vi "Main_19A_X1.vi"() -> ()   [LabVIEW 2024]
uses:
  Cluster_Towel Data.ctl
  Cluster_Design Data.ctl
  ENUM_Stripe Select.ctl
  Cluster_Design Towel ID Data.ctl
  <vilib>/Utility/miscctls.llb/LVMapReplaceAction.ctl
  Utility/Universal Utility/TypeDefs_Utility/Cluster_Row-Column.ctl
  9e3f57c0-2ef8-4495-8287-c6a42a5fb955.vi
  Utility/Universal Utility/TypeDefs_Utility/ENUM_4 Directions U-D-L-R.ctl
  Utility/Universal Utility/TypeDefs_Utility/ENUM_8 Directions U-D-L-R.ctl
panel:
  out "Invalid Designs":T1[](array[typedef])
  out "Valid Designs":T1[](array[typedef])
  out "New Design":T1
  out "Design Updated":bool
  out "Current Towel":T4
  out "Current Design":T1
  out "Towel List":T4[](array[typedef])
  out "Target Design":string[](array[string])
  in  "Select Data":enum32{"Example", "Puzzle"}(tab)
  in  "Example":string="r, wr, b, g, bwu, rb, gb, br\n\nbrwrr\nbggr\ngbbr\nrrbgbr\nubwu\nbwurrg\nbrgr\nbbrgwb"
  in  "Puzzle":string="wwubu, guw, uguggg, bgr, rgbrg, bbrb, rwgru, bwgr, uwwbuw, rwrbrgb, ggbrbuur, bb, ugu, grurrr, gbwbwb, rgbrb, bgrwrbu, bgb, wrwu, rwwr, wubr, bug, wu, brwu, w, grbw, uwbgg, gggwrggb, rurgr, uuw, bbw, wbg, bgw, ugw, brb, uww, buww, uuwgr, buu, rrbugw, ggggbgug, wwwrbbr, rgbbr, ugrr, wgwrg, bwuubub, uugg, bbrgg, bbugw, wuuwb, uwr, bugww, rwrrbbr, ugwrrrb, ubbr, rrwbgg, wb, wgr, gbrb, gwgg, rbg, bub, brg, bubr, ugggw, uuugbbb, grbug, rbww, rg, wgwwwwg, wgb, brugbbb, wgrww, bbrgrurg, ruu, brr, grgwg, wurbb, bww, ubwgr, bburwurb, urrrrbb, rgg, wwww, gbgw, rbrb, buw, wur, ruugugb, uwugg, rgrrugub, ggg, ggr, wrurr, bgg, uuru, brbg, rrbb, bbr, gbbu, grug, rwrrug, ggubub, ggrgg, uu, grb, rrrwwbg, ubbg, wgwwrgbr, rbug, rwrgwbrb, wubwgu, rrw, ruw, rbwubwgr, wwugg, bbbu, wgwr, rwgb, ruwg, rrrb, ubw, rwgw, wbr, uwgrb, rbwrrrru, guwbwg, rgbwr, wbu, ubgu, uruug, urbuuruw, rug, wg, gugbw, brw, wgrb, rbwu, wrw, bgggr, rubu, ur, uggrur, ggwbbuwu, gggr, gwu, bbwb, rrru, rubgb, wub, rgb, rbur, wuwbb, rbb, bwb, wwr, wubrwb, bwwwg, wwbwww, ugrrurw, grg, gwuw, uwwww, ubgb, gwr, gwuurgg, grwuu, gbru, rbbrrg, r, rgbrrg, ugrrubr, bw, wwbwbg, brbwbwr, rrrbg, rggb, bgwu, rrgrwwb, wrgrrb, grw, ubu, wgrugw, bbrugug, wubuwrb, gbrr, rrbg, bbg, bgrwg, urwu, uug, gruruwb, bur, rbwrguw, gbbuw, wubbr, gwurrw, rurr, gwrubb, wwwrw, wrwrbbr, ubbru, gbr, rwg, rrgwgr, ugrwwg, wwbgbr, wwubuwu, uwbb, gggbb, bru, uwb, bgru, wgu, gbrgr, urrwb, ub, u, bgrug, rrwr, bguug, gwbb, uuu, brubwg, bwrwbu, ruggur, gggww, rgu, ug, gur, wgurgwb, uuwwb, wbwgr, gbrg, rru, uuwurrr, rbgbw, ubgwgw, wgwbgu, brbwgg, uwwgw, rgww, buuu, uwu, wrgug, gug, rr, gggwb, bgu, grwg, wrwr, uub, gbuwwrwr, bgug, bwg, ubg, urrb, bbgggw, uuurb, ggw, wgrbwrg, bguw, brrrb, gwrbr, brbw, ggrrbu, uru, wrrbg, ubr, ggrr, ww, wwbgwwr, bgrr, wugbrwg, rrrrg, rww, wrbg, ubur, gwb, rgw, bubgbw, gbb, buuuuur, wwu, uubwww, buwg, ugbg, wgrwbub, wurwuu, bbu, wuru, ggu, wguwgr, gbw, gub, grr, rubgw, urrurb, wbubrr, grgwwb, gbwwru, urb, ruuw, urr, gu, bwrbwg, wrr, wru, wug, wbuwwwwg, guugu, brwurrb, brruuw, wuuuu, rbu, gwg, bgwg, rgr, bbrw, bu, gbbg, bbub, bwr, buur, wrgg, wwuurbug, bgbu, ruburubr, bwurbr, rbr, wgw, gwwug, rruu, wubgg, bwwg, wgwbwu, gwrr, wbbrrb, rwbgbbbr, gr, rwuw, rggbur, gbu, uggb, gwgr, guggbuu, gugw, brgww, wuw, rbubgbu, wgwbrb, g, urbb, gb, gbwu, uuug, ggrbbw, wbrrww, wbw, ugb, gbg, ugr, ggwww, rwr, rbrbw, wrg, wwbr, uggu, rrg, gwguuuuu, bbwuur, rgru, bburww, bbbg, wbb, uuugww, bwgg, bgggw, rugbr, wugrbwr, urw, bwu, uur, gggwrw, buwr, rrr, wwb, wgbw, urg, uwgbw, gru, bgbgurw, rwrrgbub, rwrw, buuug, wggbrgw, guu, bruuubw, gw, wuu, rrb, uuuwg, uwbugu, ugbbrr, wr, uw, ruwbw, wwg, ubru, guub, wrrwg, www, bbuuuw, guruub, wwbrwu, rwgbuu, rguruww, bgggrwr, bg, uwuwr, ugwub, ubgbu, ubbur, rub, gww, rw, urrbbbbu, urrbb, wuwu, ubuggww, bbbwg, ubugg, grgb, rwu, rugbug, ugg, wgg, gg, ru, wruw, wrrwuw, rubg, rbw, rwgwr, uuruu, ubb, ggb\n\nuwgwguuguruwggwbrbwurruwgwwwurgbgwggwwbbubgugguuurgugugwu\ngwwggrgbwbbguwgbguubbwrbgurgbburrgbwruwgurgwgguwbwgbgrr\nrgggbwgwgwuubwbwrrbrrrurwuwurgubuwrbwrbbbbr\nrguruururrwbbrgrbgrbwggrubbggbrbrugrgugggurubrbuuw\nrruggbrruruggubguwrubwbwuwgrwrguuurbrrbbbggbrwg\nwbwurbbrggubugbrgrrbuuwubwurrwururgbgbwurubbuuwbuw\nbrbwrrruwrrrubrwuugrbuuwuuwrwrbrrgububwurugbwwrb\nrbbbuurubwubbuguggrgwgwgurburugugwbgbuwbwwrrgugg\nwrbbugrwgwubgugwrruggwwggurrwuugrwrwbrwgrww\ngbwbugwgrubbbbburrbwugbwuugrbbwrrwbgrwubgwgbbb\nurgrwbruurbbururwrwwbbubgwbwurbwguguwgrbrgugugwrburb\nwubuubwggrgwgbgububrwgwbbubgwgbwwwuubrbbbuwbr\nwrrrrurbwubwuuggwguuwwwububrwrruwurrbbbuubggwgrgwugwu\nbrurwwrbbuwgugbruurgrrgbuuwrbwrugurrwrurrrbbwrwbrrgrwuwg\nurgwuwwbwwrbbwbwgwgrrbrwgubbrbgwububbwurggbrgrggbrggrrrwgg\nuugwrbwguuwwgbwwwburburbwburwgwguwggwggwbbbuburrubgbbguugg\nwbwbguuuuubwwbwgrwbwgguguwgbbggwwwurgrwgrgbgggurbuwugwrbu\nuubwuwuuwggbbruwuwbwbgwbwrrguwurubbguwwgbug\nbwwgwwubbrrrrwuubwbwrruurrwwwwggbgbrwububwwurbggwuwbgu\nbruwgrwwbrwbgruubwbbbugwrbbgwguuwguurbrwrb\ngrbgwuwwrbgrwgrwurrwbbuwwwwwbrbburrbrwbuggrgwbwrb\nwgggrubbbwwgwgggwruururugbrguburrwuwwurgggubrbwwgrwrb\nwurbwrwwugrgrgruruuggbbggubwrurbrgrbwwrbrrw\nuubuwwurrrrurubbbrrugugubgbruubbrwbuwugrwwgwrrbrwggwrb\nggbuwrwwwbbrgruugrrbrbuurwgurwgubrggguwbubrrbbwgwrb\nugwgurwrwwbrrbwrrrruwbgrwrurrrrrgugurwbuuubbubwwbgrrrbwrb\nurwrbbrbwgurbuwrgrurgwggubbwubuggrgbuwgurbbwwbbwwubwrurgrw\nbbugbwrwrrrwbgugbgguuwwbrwbbwgurubrgugrgwurrbb\nuburggbrbuurrbbggububwbuuubgwrruugbrrbuuwb\nrrwuwubggwrwruwrgrrwrwubwwrbbbuggbrggurubwubwbuggwu\nrwwuuubguwgwuwgwwwggwbwrubbrguuubrurbwuggubwbruwrb\nruugbuurwwwwrwuwurrrbrubugubwrwwwgbwbrbgbwb\nwrurbuuruwrbwgrbgbbwgwrwrrrwgwrurbrbuwrwwgbgwgrwgu\nbbruguugubrrgrgurwwggwurwbgwbwbbuugwwrbwubwgrwrb\nbbwgrrugwgrbgwbbugugwuubrbrbrbbrrrggurgbbwwuwrbbuwbgw\nrbgbwburggggrbwubbrrrrggbuwbguggrrbuwbgugbbrgwrb\nubgwuwbbgbubrgbububwuwbbbburwurbwbbuburwrb\nbbgubwgruwbuwbwrwrurbrbrubuwbgrugwbbggbwgrwrburguggwwg\nuwuubwuwgbuurbugubbgguburbugugrrwbrrurgwrwgrgbb\nwwuuugrwuwurbgwwbrbwguwugbgrbgwwbgrgbubrrgrbbgwrggwgrwgruu\nbbbwurgwwbwurwubbugrwbwbgbwrbwrwububbgbgurwwruwrwrrggrugr\nbubuwbbwrgrwuggbgrgwbbwruubggubuwguwgrbrrguwgwubbbbubugw\nwbwbguwgbrgwgwrrurwwrrrgbrwubrgwbwguwbwwuwgugwgrbbubgru\nbwbrbwbrbubbwwbgwwuwgwwgggrrgwbubbubwwwugrgwgr\nwgwwwwurwubuugruwbrrguwgubwwbuuwruugbwrubr\nrgbbbwrgburwuwwbwubwruubgguwbrbwbwrwurbggbwbrugwgrubrgbbur\ngguwwggubgrgrgrwuubruuurubrbrruwgrrwrwuwgrwwburwuwrg\nuwbgrrwbbggrwwgguwbbgbbrugruugbgrbuwgbugwrb\nguurgurbwbbrugrbuugbgruwgburwrwwrbgbrrrgbwbuwrb\nuuwuggwrwgbgbuguruwrgbrbrubgrgugwbrugwrgubbrwuwrb\nrwgguuubwrbbrbubbgwwgrgbbrrrgggbururgwgbwgugwgbgbrbbb\ngrwwrwbbruwubgbwuuubwgubguruugubbwggrgurrbwurgubbggwb\nbwuwbggbwbgwbruuggruurrwrwgubbwrrubrwwbgubguwrb\nrbwbbrgrwgbgwgbwrrurgbrwgwurrwbrwwuwrgugrbgrugrgubbwrb\nwbbgwgbwrubuwgurwbwbugwguwwwgbuwgruguwbgbgbuubwuwgwubgrbww\nuwwbwrbubgbwwuwwubbgbgubwwwgwugrgugrwwwgwbubrguggbrgrbrgg\nwbwuwgrwwguwgurwwurwubgwuwugrbbggbrruuwbgurrru\ngbugwgrurugwrrggbrbubrugggwggbubwbwrubububgbwrgwuurugwrb\ngugrgwugubwuwbbbuurrwwrubbwwwguguwwbbruuugbrwwwuwuw\nrwbbgbugrgburrggrgwgubggwwruuggubururggrbwrb\nrgggggrbbrgrrugwwwgwbwbbrrbrburbwbwwrrgrbuugrruwbbuwrb\nubbuurgrwwwuwbwwbgguurbbbgwbuugwgwuggrrbugguruwwrgbgggbbuwrb\nbwuruwwubgubbggrruwgbbgggwrruubgurbrbuuubrgbwub\nrbubbggrbwbgwwrrbbggubwwurwgrgwubgrgrrbwrb\ngwwbgwubrububgwrurwgurbbuuubwugggbrrwuuwru\nwguggrbbbwgrbrwwggrurwbggwgbrgggrwggugbrgwgg\nuuguuwwrguwrrggugbwwgwuwrguwbguwuurbwbwrggwguwrubwrb\nruuubbgrgrrrgbbrbgbrbubgbubwguububuugubgrugbgrgwrgwrwruggw\nruurrbwrbgubbuwggguwbwububrbwgrubbwgugwrb\nbbgbugbrubwggbrrwwuwrwwwwrwbgbbggrrwbguwrbwrb\nbrbugwrwrbwwwguwrgrrrggugwwruwburugurrgrurbguwguwwbrubu\nwbwubgbubwwgrrggrbbgwruwrrugwwrwuuggbuuwburbrugbguwrwrb\nuugbuuwwburgbgruuruguuuwrbwurwggbbwrrbgrurbwub\ngrrwguwurwwuwgguuugurwrgurrwgrgugrurururwrb\nwwrbuwwwwrbbgwgwbgrurburbbwbgwuugbuwuuwwuuwbbuww\ngggrbrwrugrrurwugwgbgugrruwrrruurbwuubbuuruuub\nrwuguwurugbrububbrggrwrwururwuwuwbrwwgurwgrrrrbrururrwbgbwrb\nrwbbgrbbwgbrbbgugggwwububugrbrgwgubbggwgrgrbrrbrgwwuwg\nwururwgrruuwrgrrrwbruubuuwgbrrwbgrrbbbgugbgrrguugwg\nuruwurbgrwrgwbrbbggwwbgwbgwrbrgrrugwbwrwwbggbrgrugwrb\nwrubuwbugurguuurugburubbrgrurgwugwwbbwuwrb\nbwrwgbwwbuuwbwgbwbbbrbwgwrugbubbgubuwrrwguurgrurwwwbwrb\nrrwuuwbruwugwguurgubwrgwgwgburbrwwwgbubwrwrgggrwugurbrrbu\nrrwgrgwwubwgwbrubwurbbrgbuguwbuggbrwrururrubbwburw\nuubrgrrbgguggwrbwbwwwguwugugbbuubgugrrbugbruggrwubu\nuwrrubgbrrgrbgrrrgbrwgwgrwbwgugguwwwgruwbuwwrb\nwbgubgrbrrrwbgrbrwrggugruuguugubbwrrwugbbrubrrbuubbwrbwrgw\ngubggguubrrguwrwurubwwubbugrwugwugguugguugbuwwwwubgwgbwwuu\ngwguwggwgwbrugwbgbgruwbrwgbgrwbgubbbgwgwbggrw\nwwwburgwwurgubugwrubrggbgbrrbgbwgggwrggbwbbbbubrbuuw\ngggggubgburbgrguurbruuruguwubrrrbruruuguwwwgggu\nbggruubuugbbubugwrrbuuwrguggrwrwurubgbwwwbuuuwgubguruw\ngwgbrgburrbbgrwgrurguuwrrwgggrbgbbgwbbbwrgggwbrbrgwur\nwbbbbrggurwuugbruubrbwgwgurbwuwbrbwrbwgruwrwwgrwurwuruwrb\nbbggrguugwrguwbgruwrwbggurbguuuubgrurwbbgurrbgguggubw\nuwrrwbwubbgwbuwwuwurgwurbrruruwuwguggrwbwwurwwurgbgu\nubuubuwrgrwugguuubwwgwrruwwbuwggbbwwrrwbrgbuugugwwr\nrwwbbugwrwggwwwuwwbgwwrrrbggruruburubrrubggrgwrb\nbbgbrwgwrgguwwrubgwbgubuuurbwwbbbbuggbrgbwrb\nubugbuwbrguwwbrgwrgguwwburgbuubwwgbgrbrubgbgr\nrubwrrgurbuwbrggwgbgwbggwuwrbuwgbgubrrrgrrwgbbg\nubrbrrgurwbgbbbrrrugbrwwgwugbrgbugugugrbbggrwbgubbbuuub\nwuwgububguurguugwuwbuwubgruwbwuwbubuwburbgg\nwwrbgwrgwubwrgruuggwbwwbrbggurburgrggubgwrrgrgrgbbrbgwwuuwrb\ngbgrrbugugwrrbuwrubwuwwgggwrbwwrugbgbgrgrrruw\nbwwgwruwugwrgwwburrwrgwgubbrgurgubrwwrggrggbwwgrguuwww\nrbbwurrgrwrbuwruwuwuuwrgugbwrgrgruubwburbrgbrubgrgrwguur\ngwwuurbugbgwuggwwwwwbwgrrbbgrgwwbwgrggrwrbugwrwrb\nugwrbrgrggwbwwuubrwubuuwwurbbbbwgggwgurbggw\nbbwggbubgwwuurbuguruwwbgggurgwbgrgrggwurrrrurgbrrugrgwgww\nuugwuwubrurururbggrrgurwgwgrrgwwgrwurwrwurwgruu\nuwgbwurruruwwuwgbbgwwrrwrwbwgrrbwbrwgwbbwubrgruwub\nguugbrrubwbrbgwrwwrurrwwgbbgwgwrbuggurgruuwgrub\ngbgurwuuwubrrugwrrugwbbbrwbrwuggrwrrugrwbgu\nbwguugwwwuruguwrrwwbbuguugbggbwbubbwgwrgbbguguruwguwuru\nbbwrbrguwrwbrgruguuggbgrbrruguubbuwwgrbbuwrwwgrbwb\nbuwbwbbrurrbubrwgrgwwwbgburbruruwbbbubwrbuuwgwwbwu\nurgrrrurgwrggugwbrwubgguguuruurubbwrrrwrb\nbburwruuwbugrbwruuuwguubrbuwuwbgbgrbubuwbgr\nrbgrugguurbrrbbwruuuuwgwrggwwurbbrggwrruuuurgggbrbrbrb\nrguwurugbwbwrbbggrgbgrgbwwuwrbbubugrwrgrrrbbbrburgubgurggwrb\ngwuwuuwugwgguubruwwrubrurwrgwrbbgruuuubwwurrugwuuugwubg\nbgubgwwbrbrwruugbbbbbwrbguwbgwgubgbbgbbgurgrurgggugbbwbr\ngruwwbwwgbbwwbwgwgwwubwwbwubwrwrgurwuwgrbbrurgwg\nguguwggbbbgbggbrbrgwbgbrwbgrgruurwurbwggbuwug\nrbrbbuurgbgbgbgggbrrwuwuwgwbwbwwuwbgubbbbwr\nbgbuwugbugrwwwwgrbbgguwbrbwuuwgrgggrrbgwbwgruggggwwubbwrb\nggwuurgbwurbwubbrgbbubgrwguwbrwbrruwgwgbrwgrrurggwub\ngggruuubuwrrugggruuguubbrbbgbruubuwrurwbrwggbrgrrburwggw\nrrugwrwbrgbbwrgwgbbbrwrgbburubggugrwggrbrbwubrgurgbwrb\ngrbrubguwruuwggbwugwwgwuwwggubuwuwwrggbrbuurwubwbbwrb\nuwbwuwwbbrguburrwrugburgrwuruwugbburubwguugwwru\nuuwwrubggwwwuugrgwbwgbbwrrbburuguurbrbwuwwrbggurbbwguuw\nubugbwrguwrrwurwuwbrbbubbbwbgugwgbrbwruwwwrububgur\nggrrburgrgburuwrrubububrrbgruuguuuwwwgwwrgbruub\nggbuugwurgbgrwggurugubwggbbbubrgurrwwburuggrrrgbbbbwg\nggbrgrwuuwwbwbuwwwwgguwbbuwuwuwuwrwgwwubwwuwrb\nwrbrgugwrbwrwguggrrggbguwrguuwbwwrrubgbbbuwwrrbrg\ngbwbwrgrbwurwuggwwrwwgwrbbwrwwrbrrrrbuwuurrburruu\nbgugggbbburbbbrguurbgrugwwgggurugbuubuugubwrwr\nwrgbrrrbwwurbgbgbwbuuwbwwbugbgbugrwgwuuubugwrggwwbbbwggwgwrb\nwwbwbbrwrbruwrurwurwggwwbrbuugbugbrwgubggrr\nbrbubbburuwgrbuwwuwrurrwwubrwugwbgburgwrggbwuwrguwgwuu\nrwurrbrggrrgbbgbuububrrwbguwrgbwruwgrrruburuurwwrwbuwgbbr\nbwggbuggrwuubrrwubuwrgwrbuwwurugrbbguuwrrugbgburggububww\ngruuwburbbgbrbwgugwgwuurgububuwugguwuwwrbw\ngrrbgwbwrbrwgwrwuugwbbgrrggggwuwgwugbbgugwbrugwbwu\nrugruggwruburugwugrgwbugwwugwuwrrgrgrggubrgbwgwwwg\nurubrbgbgrgwwgwbrgbbwbrruuruuruuururggubwr\nburbwguggwrggrwggubuurrgwbgwggwrugwwuubgrbwbgrrbug\nwwbwgrrwbwwbrugrbgwgwgrwwggwbrbwbgggguuubwbgbburguggub\nurrbbbburgwbwbbwrgubbggrwbbubuwrgggubggwrb\nggugrbggurrbggrwruwgrbrwgwbuurrgrwwwgugurrrbwgbbrbbggwrb\nbwgubwruwrgbrbwgbwbbgbwbgrbbruubbuugwburwrb\ngwrbbrwugurrbugrbgruwruwrwwguwubwubwbrwgrruggrr\nrwgubrrugrwwwubrwwwrbrwwrbgruwgrubbgwgrwrb\nbrrbwgwgwggugbgrrrrgggubbwwwuururbgbrwugwbrbrbwuuwru\nurbrurgrbgguguguuruwurgugwwgrubggbgbwwwgrbugubwggr\nrbgruguwrurwbgwgurrwrrrggugrwwbrbrbwgubuwubruubwrurrgwbgbwrb\nggbwuuuwggggrububwwrurgbrbrubbwgbbbgbbbgbwuwwgggbwrbuwrb\nrbbbburwggwurrrrbggwgwwrurubwbgbrbruguwwrwrgggrugubw\nrgwgwwrgbrgrwgrrbrburwbwuugbgrwwwggrwrbbwrb\nubgrwwwuubwwwwgbbrurbuuruuurrbuwggbbuurgrrwrgwb\nwgwwuruurbgwruugrwgrbugrbbwbgwwgguubrwrrbr\nbwrwubggwgrrubgrrwuwuuugruuuubuwbrbbwrrbgrwugwgwugrguwrb\nrguwgwugururbwwgwwwgwgwbugubbrbrgwrwgguguwbwruwrrrbgbu\nwuuuugurbwrgbuugbrrwgggwwwrwrrrrgwrwggwrbb\nwwbwbugrwbbuwwwrwrrrubrbgwwwburwgbgbwwbuwrwugguurbg\nubgbuubgrrwruwugwbwbwbwwgbwbuurwwuwbubwrbug\nuubgrgrrugubggggwgrbgbrwrwbrgrwbbwgrburrbr\ngbwwugwbgggrbguurbrburbwwrugguwbugwwugbuwwbguu\nwuwgrgrgwgrbuwgrbgburuuwrbwguuwuruwgbwwubwwbururbw\nwwrwgugurwrbbbrwbwubggguuwrwbuurbwbwubggbbuurrwwbubuwrg\nbburgruburubrbwrwwwbrgrbuwgwrwggurburubrgwgbbruw\nubrwbwubbbbwbwgruwuuwbrgbuwwuwuurrrwrrrwgb\nwwwwrbrrguwugugbgrggrubbrgrurggbgbuwwbrgggwuguwugbrwg\nrbrbbuwrubbbugbgwgurggrgbwrrurbburwrwggruwrubgbgwwuuu\nwuuugbgwgggburrrrgwbubbbgrubbgburwrbugbbwbwggrgrg\nrugwgubuwurrguwbwwurrggrgrurgwbbwbubwwgbgrubruuuwwbu\nbgburwubrrwburrbwgwuwwwwurwuuwbgbgrwggubuwubwwggrwrb\nuurbururruggwrwuwbguwwwbbwrbbwrggwrgbwwugwrwuwrw\nbburugbugwwwwggggwruwwggrwwrbrrbwgbbbuwgwgbwwwubgrgbwrw\nrgggubrrbgugguwwuuwurgubgwrbuwubwburwuubrgb\nrwrgwbrbbwrbuwwuurgwuwwbrbrwuububrgubbrbwrguruuub\nuuugrguwruwwuwuuwgbbrrwwgruuwbbgwguwwruuwrb\nbubbubgwwuurgwrbuuurrwrwwrurwgbwugguwgbbggggww\nuwruwuguubrrbbggbgrbwrwwwbwwwggggruuuguuugbwrwwrgw\ngururwuubwbbugububgwugbugguwuwgwrugbrwrwrb\nwrrbwuuwbwbubgwrruwgguwgrbggubrgbgugrrgrubwwwbwbr\nrbgwbgwububrrrwbuwwwwgrurwrbwrgurwruggguggurrrubbbwrwgww\nwggbrggbrrgbrrgrggwbbwurbbrgugugrbrgrwwbrgubwrwuuruubwugwrb\nrrgbggurbrwuwrgrbbwwubguwgurugurwurwbgwrrbbwwuwwbg\nwbbggrwrgruwgrbrgburwggrrbbbguurgubbuwbruwwrggrbr\nwubugrwrrwuuugwuubgrubbbbgurguwgrwgruwwruguburwuwu\nwbwuggubbrwugwbwrrwurgubuurrrubrgwbruugrgbrrbrugbwrruwuubwrb\nrrbuwruwguburwgugrwgwuguwuubgurggrbuugbuwrb\nwrrbuwggurrggwubgwwuggbwuuwwurrrwwrwurrburgwbwugrgbuwwrwrb\ngrrurwggwgruwrrbbwuugrwgrgggbrgubggbugugrwrb\nwwwrwbuuwgbugbwurrgwuwbuuwrbuurugurwbuuuburrurwrb\nruruggbgwbggrwwrwrbrrgwuguwwrwurrguwugurbbruwbrwuu\nuwuuggwurgbwrrrbruwrrwrurgrwrbrwugrwbbburwurbwbru\nrrbwuwgrwuugwguugbrwgubrbubgguwrugrwbwrrbggbgrrrugrbbgr\nrgggrbugbubburuwwbrrrbuubrrwubuuuwgbgguuuurrubrwwuwwugrbwrb\nurrgwwwrgwrrgurrgwbbrggwrgubwgwwwugruuubuuwggbuur\ngbuguuwwrbggrwrrubwwgrbwrurugrwrguuuugwgwrrrgubgbwb\ngwugrrwrgubuwggwrrguubugwrbururwgbwgbbugwwwrb\nbruuwuwbgrbrwbwwubrbbwrgwubgggwugbuwgbrwbbwruubgwbbrwwwubg\nwwgurbbbbbwbwwrwguwbrururbwurgbgwurrurbgur\nwwrgwuurruwuwugbbrwbwrbbbuwgwwububrwwgggbguwrgwrwrrub\ngugwrrrwugugruuwrguwbwwubbggrwbgbwrugbuwrb\nrgubwgbggwbbwggwgggrrrgggbuwwrgrwggggrrgwr\ngbgrbggbgggggbgugwgubggwrwwwrwgrbrguwuwgwrbbrbuwwgrwuwrb\nwwbgrrggrbgrbwbrrrbwrwrwbwrbrrwbwuugggwrb\nwbbwbwbgrbwwwuguubbwgugrugbbrbbggrwwurururwggw\nuguwrggruugrgwwuubbrbbbgbbgugurruwruwbugwrugubwwbgbwg\nruwbwbrubggruwbrwrurbrrrbgrrwrrgbubbrwrwurwuubwbrruburwuwrb\nugrrbgbbugruruwbgbbbgwbuwgbwugurbrwbgurggbubwwrbb\nwbbwrwrwgurubwgbrgwgrgggrguruubburrubwugggrrwgbbrugw\nuugwubrgwuuwbrrrbgruuwruwwbuuubgwuwwwuwbruguuuwgrbrwrb\ngugubrrggwbuugubrbgwgbubwwgrrurubwwrbbwbrgrr\nwrggwguuguuwbgburwwgwgwbruwrgrrwuwwrgbgugurwggbbg\nwwuugbgggubwwwgrgrbguguwgwwwgbuwgbugwgwwguwrug\nuwuurugbwgbrrbgbbuuwuggbrbrwubwbrggwbgrubbrrggbuubu\ngwggubgwgubguwrbggbwwgbuurbbuubuwwugbubwbgbbruu\nbbubugbuwwgbgubrbrguwggbbugggbuwuubbwgrwgwg\nrrrrwugwuurrrbggrbwbrbrugbrbubugrbubbrguwwwwwrrgwgbuugbu\nwrurguruugbwrwbgguggbwruwgbbwgguurwbgubwruuwru\nrwbbwbrbwuwrubgbgwrbbuwbgubrgbwrrwwuwgbrwgurgubburuug\nggwubrwwuggrrwbuuubwwgbbgwurwgrgwwuwubbrgruurugwuguggurg\nbbrugurbrurbgrbubwurrubbrbbgugwbbbwuuuwrb\nwwgwwbruuuruwggbbwuuuubgwbubrbgwbwwuruuguw\ngburwbwbgrbwbgrugbuwubgrrbrrggbuwwrwrwbguuuu\nuwuwgrbggbrwgwggwwgbrrwburuuguwbbwwwrgurbgurrwgwurguwrbwu\nrbwrbuwrwgbbwwggrbwbwwggrwguwggbwrgbrrubgubgugwbrruwwrb\nbbuggbgbwgwrrrggbubrggrurugubuwbwuguwbugrrggwuwbwrggbwb\nugggrbwgwuubwwggggwuwwwruuugrrguwwbwubrrwugwrrurwgbg\nbwgrgbubgbuurggguubwwrwgbubgrrgrgugwrguwruwbrbwrwbbwbbbb\nwrrrbgrbggruggbbuwwuubrruwgbuuubgwbguurrubbubb\nrbwrrrrubruuwgrgrbgwwwurwurgwbugrbbwwgggugbu\nugbggrgrguwwwggbruuruubwwgbwuggwbrwbwwbrbwubrubgbrrgwuwrwrb\nrwrbrubwbburrurbuwgrrrgurwgrwbrgwgwwrbwgbrwr\nwbwrbruubggrgwbbrbgrbuwwrrrbwwburwgwguubuwguwbrgubbwrbrbwrb\nrgrrbwrgwbbuuuruuwbrubbbuburguuburrbgrwbgruwru\ngwrgrrbubrwgurwgruwguurgruruubgubguggbbwwrb\nwgbbuwurburbwwurgbgbwgggruggwurbwuwbubrwrrwbburbgrwgug\nubugbggwuwguwwwuwugwbwgwwuuuggrrrrubwwubwbwrwrrugwbwrgwuu\nrubggguguuwgbuwggrruwrwrgruruguurrubwuwrgruwwgrrurbwuw\nwurbburwrubbwbwrruwrbrbuuugurbwuwwgrbrbggwwbgugubrrg\ngugruugwruwuwrugbgurguguuwwbbrwrurrgubwbwbrgbwrb\nwugrbrbgwbbuuwrrgrbwgwrruuuubrbruwggurgbrg\nrurwugugguurgubwbuuuurrrwbrrurbwruurwugrubrgubwrub\nrubgwwrrwwwgguuggbwuruwwggbrubwbrwgubrrgrwwbuwggbbburwurbwrb\nwbbbggwuwbwwgguruwguwbugwgruwwrwrgggurwwuwbbwubgu\nbgbwbbwruuugugbrwburuwwrwbbbuggugbwubrrwgwugbwguguuuwru\nrbrwwwwwgbruwguuuuubruuurgbuubrwbrbrwurgburbub\ngrruruwbrwwrbgrgbgrwuwrgwwuwbbwgrrrrrrrrrggbbbwbbbbu\nurrwbbbrwuggrggbgububbrbubuwggwuugwurbbbwbbrwrb\nrwwubggwrrbuurwwrrruuuruwggggwbbuwurrurugg\nbgrbrruwrrgrwbwruwbwbguugbrrggrbgububwbuubrububggugg\nrwruuwbuwruuwrrwgbwwrbwwwbwwrwwuuggbggwbbrbbbwwg\nrrgwrgwubgwrwugbuurgruburburuwwwbwwwwrgwwrgwrgrgg\nwgwrrgwwurrrubwgwrgbrbwgbbubrrrgugwwguubuwrbbb\ngurggwuurwwurwrggugwugrbwubggwwwugrbubwrubbuw\nuruuwurrggwbgrugrrbbubwbwwggbuuugwgrwbuuuugrrwbr\nwbbguguuwuubwwrbrbbrugwrwuuwgrggbbwurrubrrgwwrb\nrruuugbgbgrrwwrwgrbugburbubuuggurguugbwgggwrwwbubb\nbrbgwwbgrugurrgurbbwbrwubbrbrrwugwrwugrwwrb\nbuurubwuubrwbugwbbrrgwbgubrggubwurggwbrwwrrurubwrgrrg\nwbrbrrrgrrbwubwgrwubgrgrwuubbgwwwugbwruwugwwgubww\nuwrgbrubwbuubuurrrbwuguwbggurbubuwgwbwrggbggbwruwuggguwbw\ngwbwgbwbgrwbgbbbrwwggbgrurgrwguwgrbruuwbugwrbuwwbwrb\nguwbwbrwgbgrrrbbrbruwwbbuwwggbwrrbuubugwbrwrb\nwrubrurubbbuguurrbguugwurwuuuwgubrwbbgguwwbbbwwwrbwgwuwgr\nrurgbrrbwwbgwbubuggwugrubbgwwwrubuuwbgwgbgwugrrugrub\nrwugwrwwbuggwbugbbwrbwwruggbgrwuugruurgrbwwbuwwurubgbr\nbwbwuuubbgurgrgrbggrubuuwrugwgwuwggwrggbrbwubwgwguwwrb\nurrgurwuwwggrubgrrwrugbbgbbbgwrguggrbuggrgrgwrb\nwuwurrrrwbwgwwggurwuwbrrgrburggbwgrggbgrbrrggburrggwwrb\nubugrbugubbwgbbbwwgwgwgbguwwbrgbrgwubbwgwwruubgrgrrrb\ngurwwrggbbbburwbgububbrwrggbuwgbwrbrrugburgrgbu\nubgbbrrbubrrubbggrbgwbwrbrwubwuurgwbburwwgr\ngwbrrgwgubbbbrrubwgrguguggwwrbggrwrwuuururwrwguwgrbuwbuuwrb\nggbubbbbwruuggrwwuuwbbwubgbururrggrbbwgwrb\nrgbbrgrwgrruwrwbuurgugbrububrugbgwruwbrurbrwwuwbbrgbbrugr\nurruuurggrwgugbgrwgubrbbbbwuwrrwgrubrurgrbuwrgwu\nbbwwwwrbbuwubgrrgurbbruwrbrwguwrbwrurwwwbbuwgruubwwwrb\nrbrggubbuwguwbggbrrbbwrrurrrbuuuggugububbbbwrrwb\nugwgwwwrwruugwrwrbuggwuuwgbubwgrbrwwgrggrrgrbrbgbbwgwrb\nggugburbbrgrrwgwbwbwruuwugrbrrrurgwrbrrbrwubr\nububbrggggrbruugrubrwrbgbwggwrbrwubggubgggrrgbubrrgrwrb\nrrgwwwrugrurwuggggwrbbwugwwwwububgbrbguwwwguwguwrb\nuuwwwrbgrrbwgwuwrwwwgwwwrbbrbuggwwuguurwgwrb\ngurrrubbgwubwuggrrwwbbubbrgbgubruwrgubggrwgrburrrrg\nuwugubuuwurruwruubgbgbwwggbrwgwgrbbuwugwrb\nwwwrbwrbwwgbrbrwbrggrgwrurrbrbwuruuburbubguwwugggrbwgwgb\nwbgugurgwrrbbwugwbrwuwrwruruwrrugrruugwuggggw\nrwbrwwgrgwwgrwgwbgwrwrwguubuwwbguwggubwggwwbww\nrggrruwggwrrgggbrruwrgbuggbbgbwbwgurwrugwbgwwwr\ngbbwrgwwrwgguurbggrbgbwggbbbuuwururrgrgwgbgg\nwbgruwwwubrbugwbuwuubwgrubguwgwbrubrgwwwgwbgwwrrugbgbub\nugbwugubwgwbuggrurguwwubwrrurrbrgurrbrubwuwrwwwwwgwwgrwwbw\nwrwubuguggbrrbugwbwwwrguuuguubwuruugwbgwbguurgwwbggrwwbuwrb\nuuugbgrgwrugwguuuuurwgggrburwwgbwrurwbgrrwrb\nwbgwguuwbbuwggubrrwbgrgbwuwrgbubruwggbrrubbwg\nubuwbrwbbbwbguuwgugrbuwwrgugwubgrburbgbbrrgrubbbbbu\nugbubrurbgwgwwgrurbwugbwwwbbgbugbbbuggrwgrbugbgwwbuwrbuwrb\nwgrwwuugurbgrrgwwbwrubrgrrwwubgbuggwbbuwubu\ngbuwrwbrrrwrwbwwrgbugrbugbrurrgggrgwgwgrrbgubrr\nwugbuggubuggbrggubwgggbgbgbgurrgwwbrwwwwrb\ngrgugwubbugurgbguwbgbrugwbugbrrwubwrwuwrgbrugrgwrwrb\nguruwwrurwurwugbbrbwwwwubuwrwuuwwugwruwbggbbb\nbguruwbbggggbgugrbgrrrgubbbrubwrrwrwubrwgrurw\nwbbrbbrgbbgguwbruuguwbbbrbrgrubgugwrgbrrgrwruguwrb\nwgrbrgbrgwurggggurwwwggubbggrrrgrubugwuggb\nbbwuwwrwrrubruuggwwbrurbgwururwggwwrrrurrww\nubwuugrgwuuuwururbrguurgrbwwwrrwbwruwrgwururbugrwrru\nrgbbrwbbguggwbrwwbbgrburwbbwwgbrbwbbubwwrb\nuuwuuubgurwwggwwbbbgbgbwbrrgbrrwrbbuwwwgubgggbbrwbrr\ngbuurwggrrggbbrgbuuwrgrggrwgwwrwugugwbgwwbrr\nbwbrgwbrgwwubrgubbbuwbrubwrbgbrrbbbbwrwbgwguuuuubrgrgrw\nguwguururgwuwuuwgwbruguwbbubuwbrggwwugrwruruuugrwrb\ngrgwuuwrbbgrrgggbwrugbgwbbbrwuuwuwgbwugwruurrrbbuggrwwwru\nbuwggggwrrrruburwbrugrwrrgwuguwggwbwbgugrgugwwurbbburrggw\nugrwgbbwwwbbgruubgguuruuuururwwbuugbgwwrgubrrbuwwugggw\nwbrbbugwgburbgrbgrurrbwwwrbwbwubbgrurrurwwrrbwgbugugw\nugugwbwwgrrgrgbuubwrwbrrurrgbubggwrgbugwrgbggubbruubgw\nbwwubbgwwrrwruuruguugugrwgwubbguburuurwguwbwrwrb\nbrrbwugubgwrgurrrgrbbrwrurugrugwuggwrgrbrwggwbbuwurrwwruwrb\nrwbbrbgwgbwguwgbgwurgrbuurugrrgwuwuurubrbgr\nuwwbuuwgbwgggwrububuugrwurgggwgbwbubuurgbwrrwbbrwuruwrrrb\nbbgwbwrrruurwwugbggbbguggguurrbbbbuubbwbwrwbrwurrbuwgrb\ngwgwbwgguwwrwugugwuuwurwgwgbuwgbgbwwuurwwggrubb\nrgburwwwuurrgbuwrgwrbugwwgguwwwgbubuuggrwbgubrwrgwugwbuwb\ngurrbwgburruggbrbuguugbguruwurbuugbrgbguguuuubwggrwgrrwbwwrb\nruggwuwgbgguwwuburgruwrbgbubbwwugrbwuwwbrbrrwbg\nwwbrrgguwbbguubbuuuuugwbbrwrrgrruwrgwwrbbbbwgrgw\nbwbrwbwwrwwuugugugbrbrbrrbwrwrruguwuwwubbugwgurrr\nwggrwwubuwruwgugrguggugwbbggugruuggrwbggrwbbw\ngbgubgbwgurbwrrrgbuwwguwrrwwbwuwuwbgburrbgwbgwr\ngrrububuwruwrubrgwwbrrgrbwugrggwbrgbwwrb\nuguuggrrwubrgrwggububbwgbbwgrwurwwwgwbubbbruggrwbrbgwrb\nbrgurrbwwugubrrgurrbbrbuubbwwwwguwwgrwwugubgruruu\nwrwubrrwburuwbrgwwuggurwrrwbbruruuwuwuwubbubuuu\nbwbugbrrbwugbwrubuwbuwwubbbguwbrgwwurbgugrgrwgwuwwbwubgwrwrb\nbwguwgurgurrrbgbbbwbrrrwuwbrwubruuwrbwrb\nrbubgwbubuwwbubbrgwwgubgwwrrgbubrwbbrwwrbwwuwgbbwrb\nwrbbgwburwwwrgwggggrrbubbggrbgbggwurwruburwubrubrgr\nrggurrwwgururrgrwwwgrugwwbguurbbwbuwrwurrrbrggbbbbrwwr\nugwwgwrgrgugrbbbbubrwrubrbguwbrwubgrwgrrgbgggwugw\nuwgrgbugbwbbggrgrbbgrwrbggrrwbbwbugwrwbrrwwuuwrb\nbguubugwggwguuggbguuwbgwbwruggwrbgbrrbwbrrbgwrbggwrbrrbu\nrgwwbubbbbuugubwbrwuwwrrruuwggrbbrbwguwruuubgbwwgwurbgbubg\nuuwbwbrwwubbrwuuuwuwwgggwwubburgwgwbrurrwbrbgbbburwgb\nwwrrbbwwbruwbgbggbrbbgrugubggwgggugrbuurgrbbgbuwu\nugrbwbwwgggwrgbbguugrgggwrggbuuwuwubrgbruwbwrb\nubggwbwguugbbubbgbbguubwuubrbwubrubrwguwwwrb\nrugburrbwruuwrwwgwrwggrubgwbuuubugbwuurgbg\nggrwrruwggbubrurubgwrbwrgbwgwuwrbbbwbuugwubrubwuwbrbgbgubg\ngrgwugwuwbgwuuwuugrgwwguwbburuubbbgubbuwgwg\nruwrwrwwrwgwwrgbubgbrbrwwbgurrwrrgbruuwgrgrrrgurugugu\nbrbwrgurrwgwrruwubrwwwrggbuururgrguwggwbbgrgubrw\nbbuwggrbugbbgbguugwuuwuubgwgbbrgugbgbwbrubbbgugwrgrgrgruuwrb\nwgbgbubuwrurbuuwgrugwrgrbrwrgwuwbbgwrrrrwrb\nwgwrgbbbuurubgwwrgwguururrubgbgwrbgwwwwwggggbrurgrr\nuwggrggrbrruwuruwbuwurrrwwwwbuggbguwuubwuwbubrrwrb\nugubbwurwurgwwrburwuugrurguuwruwwrwbgruggwbwwwgwbb\nubwgwbbgbrugguwrggubbrgrbgruuwugbgruuwggrbgwugugwugrrwwg\nwggrgugugubgrrrbugbbbwrrrwbwguuruugrwwrb\nbwgwwbrwbbubgwubrwwwgurbwbrwbubgbwbubwgbbggrrwbbgbwrbbrr\ngurwrbbbrbrurbrrbugrrrguurwwbbwugwbubuwrwbrgbgrwrbuuwrbuuw\ngwwwwuuubuguwwurubwwrggguwgbrbbbgbububgwrbwbubbruwbb\nuwwwbbggwrgbrgrubrurwrgugrbubuwwruugbwbgubugbuguuuuurbrgr\nrrbubwbuwrgrrugubbbuuuwwbwgurrwwgwburubwrwrb\nrurrbbgurbuuruwuuwrurrwbbggrrrgguwgwrurgrurubwrwwrb\nugbugurrgggrgrbuuwgbuugrrgbuuwugbrwrrgbubbbbburuuuwww\nwuwgugruburwguwrwgwbwrbubbrbgwbrgbwruruwbbuwwwugurwgurwrbbb\nwugwbruwuggrruggrbgrgubuubgurbrrrruwrguububruubwugwwbbwbu\ngrubuwwurrbbggwbwwwruuuuubwgwubwuubuuwrrrwgrururbggbbggw\ngwgrwbuwuwgwrubbgbugrgwbgrbwbuwgrggbwrrubbuggwbgrwgbggg\nuruwrwuwbrbrwwruwgurrugrbwguuubwrwwurubgrbgrgwwur\nrguubrwwgubuwwruruwbuggbrburgrgurugwwwwrb\nuuubuubggrugbgbgwgbbgburuwggrrggwrwruwgbuwwbrgu\ngwgrgugwgbwbuwbgwgbrguuguguugrrgrbuugugbrgu\nurgrwwwrgurwwrwwwggbgubbrgwwwruwubgbrgurguurwugrgwrb\nrubgwbrwbgrruuwbruwrgwbwbguwururubrgwrurbuubww\nbrurbguurgbggwbbgwwwugbrbgwrwbrwrrbrwbugwuguwrbwru\nrwrbbguggugwwgrbrrwrbgruwrwwuugbrgurbwuguwwubgbgg\nwgrgbgbwbbggrwgrbbbrrwubgrbrbgwwururguwugbgrgrrug\ngwuurwubwwguggwwbbwwugrwgggwwurrrgrrrburguwwrrb\nguggrruwrbrugwrwgrbgurbgbrgwugwwwwbbbwwrwuwug\nuwgrrgrbbgwrggrwwwgbgbrbbrbuuburbbrbrugwurugwbburgbb\nwwwbbbwbbbrbgubrwbbrubugbrgrrrruuwgurrwwwruwgwrguw\nuuubuwgwrwugrbggggbruugbrruwuurubwwgwbwgurbgbuubbgwbuww\nwbrrwgbuwggubuggrugbwwbbbbwgwrrbgggrrrwrbgrbgg\ngbbbrwwggbugrbrrwrgbuwgbrrrwgwgubrruruurwguwb\nrrbbuwrbruwruwurbggburwwbwuuwrurbbwrbuurubggwrb\nrrubbuurrrgbrwwuwrbwgruuwbbwugrgubgbwwruwbburgbwb\nwrwugbbgrbgurubrwwwwwbbbruubwgrgburbwbrgbwbgwb\nwwrwugwbbrubugbrrgrwwbwbuwwwuugbbwguruggwgwrwgwrggwrgrgwgwrb\nbguwgugwbgwgubwwbwwrwubrrwubbwgrbwgggwuuwgrbgwgwgrwwggrb"
  out "Answer":u32
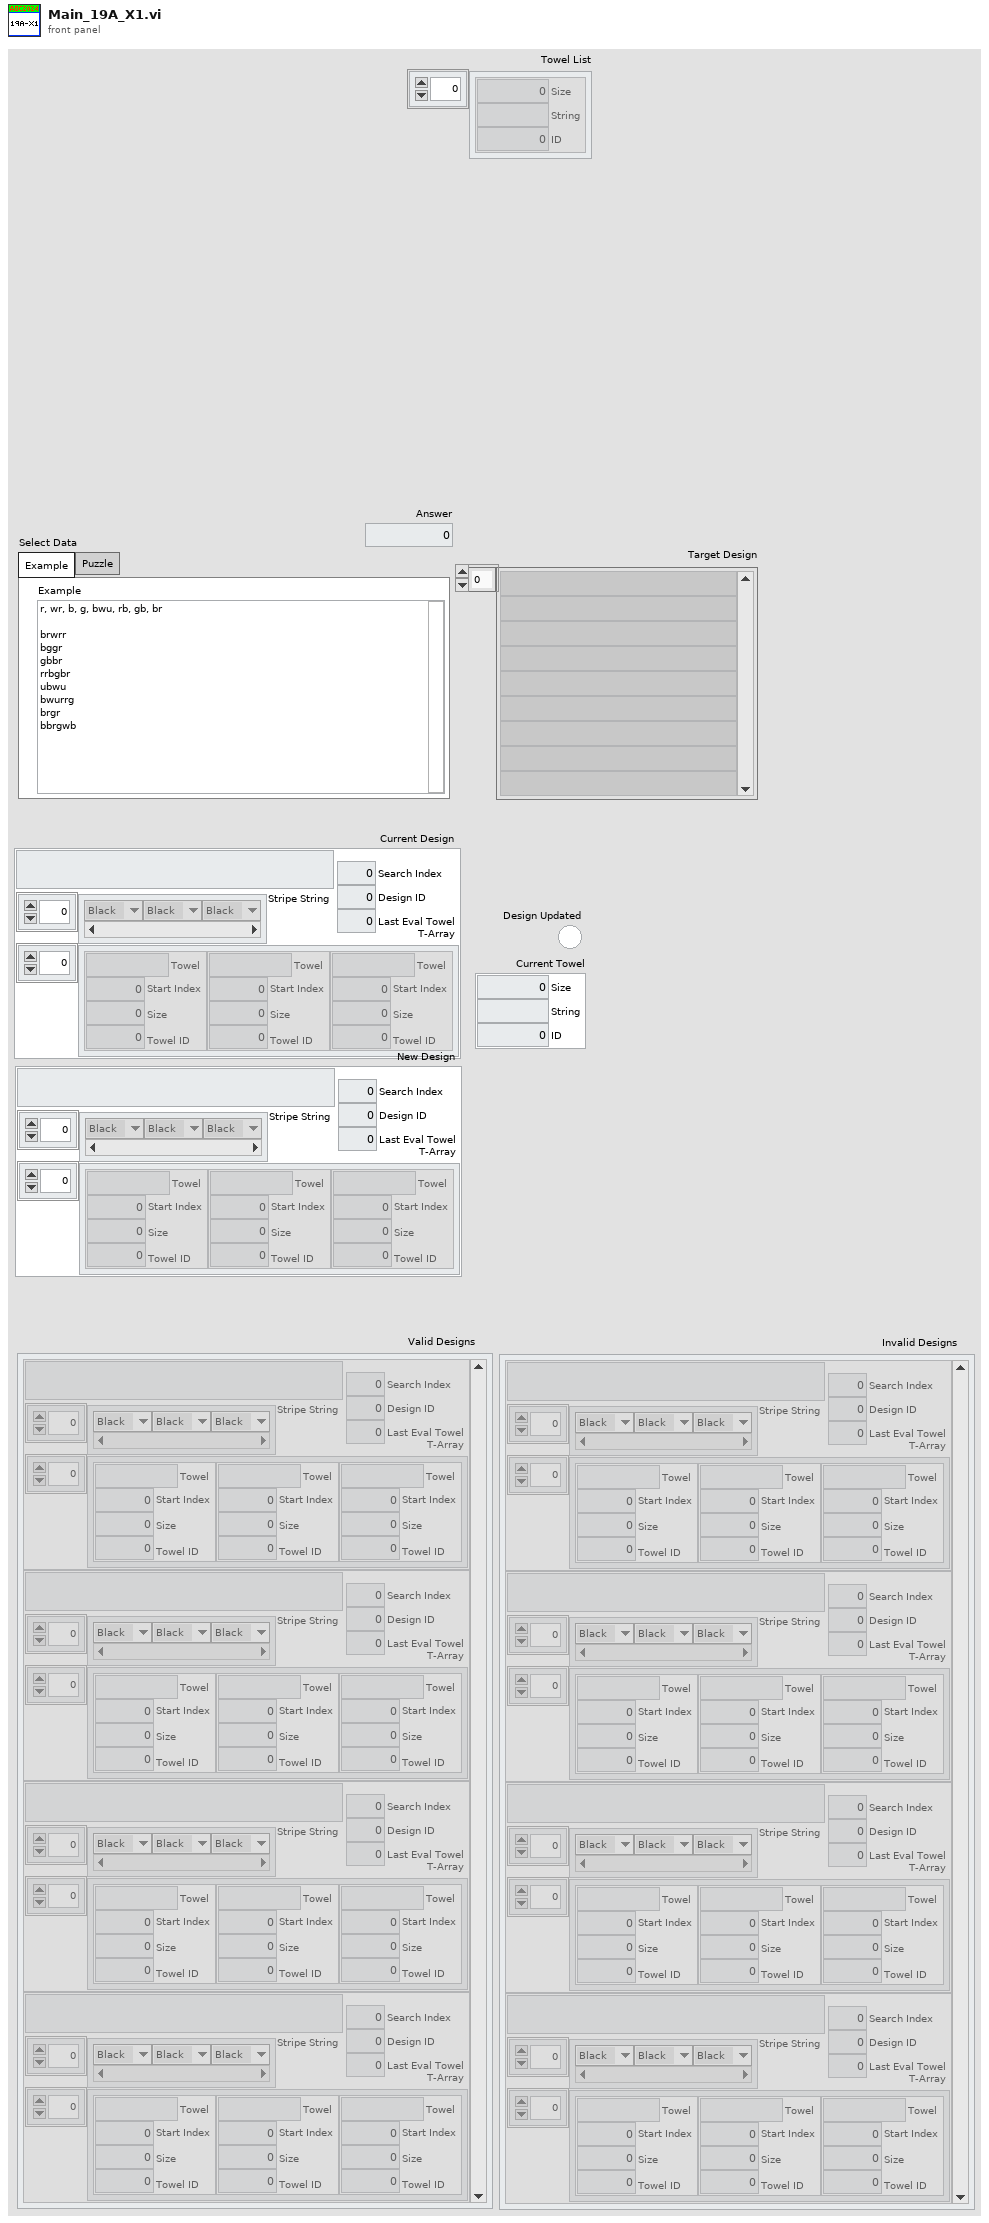
[diagram p1: front panel]
types:
  T1 = typedef "Cluster_Design Data.ctl" = cluster{"Stripe String":string, "Stripes":T2[], "T-Array":T3[], "Search Index":i32, "Design ID":i32, "Last Eval Towel":i32}
  T2 = typedef "ENUM_Stripe Select.ctl" = enum16{"Black", "Blue", "Green", "Red", "White"}
  T3 = typedef "Cluster_Design Towel ID Data.ctl" = cluster{"Towel":string, "Start Index":i32, "Size":i32, "Towel ID":i32}
  T4 = typedef "Cluster_Towel Data.ctl" = cluster{"Size":i32, "String":string, "ID":i32}
  T5 = typedef "ENUM_8 Directions U-D-L-R.ctl" = enum16{"Up;-1,0", "Up-Right;-1,1", "Right;0,1", "Down-Right;1,1", "Down;1,0", "Down-Left;1,-1", "Left;0,-1", "Up-Left;-1,-1"}
  T6 = typedef "ENUM_4 Directions U-D-L-R.ctl" = enum16{"Up;-1,0", "Right;0,1", "Down;1,0", "Left;0,-1"}
  T7 = typedef "Cluster_Row-Column.ctl" = cluster{"R":i32, "C":i32}
  T8 = typedef "LVMapReplaceAction.ctl" = enum32{"Modify Entry only if found", "Add or Modify Entry", "Delete Entry"}
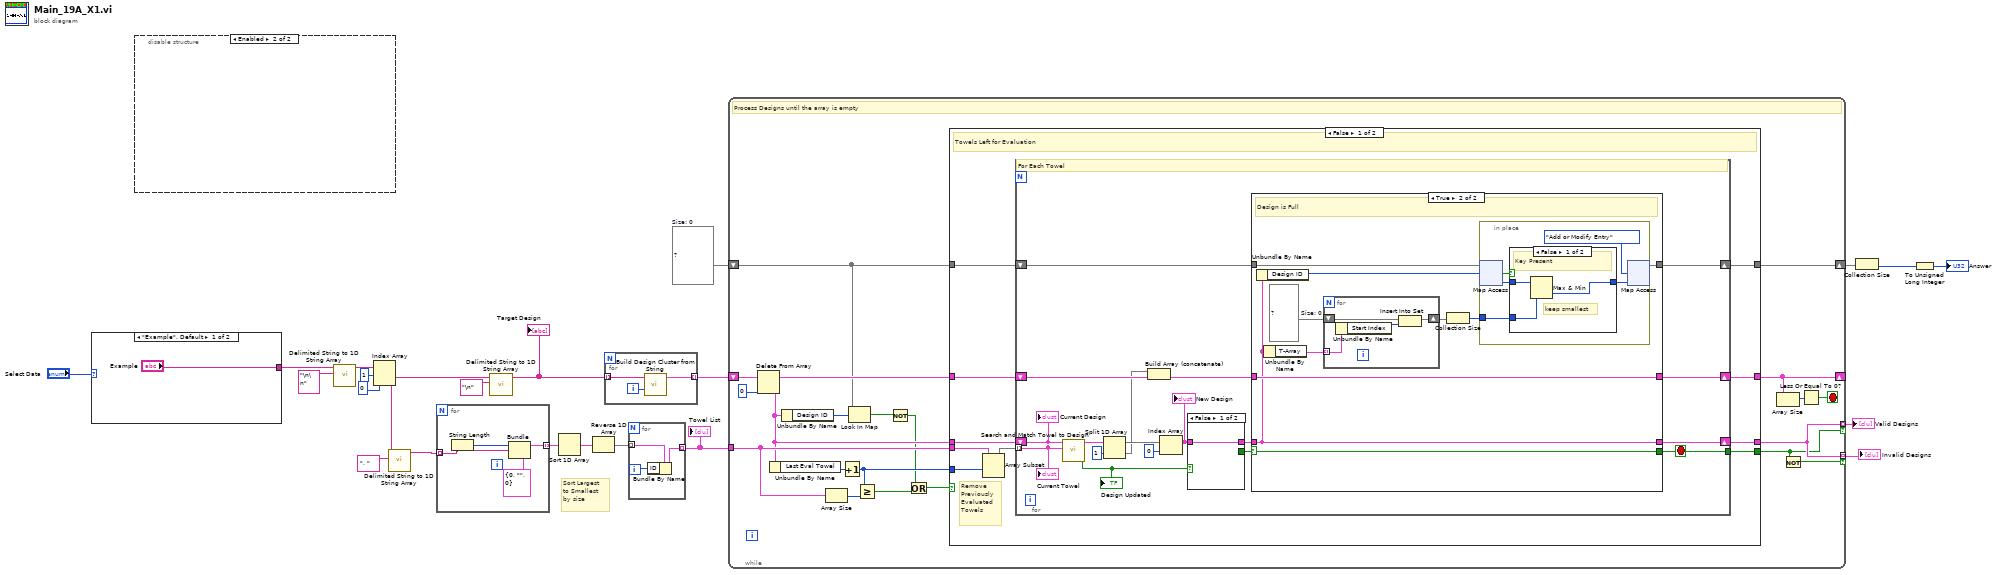
[diagram p0: block diagram]
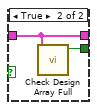
[diagram p2: hidden frame]
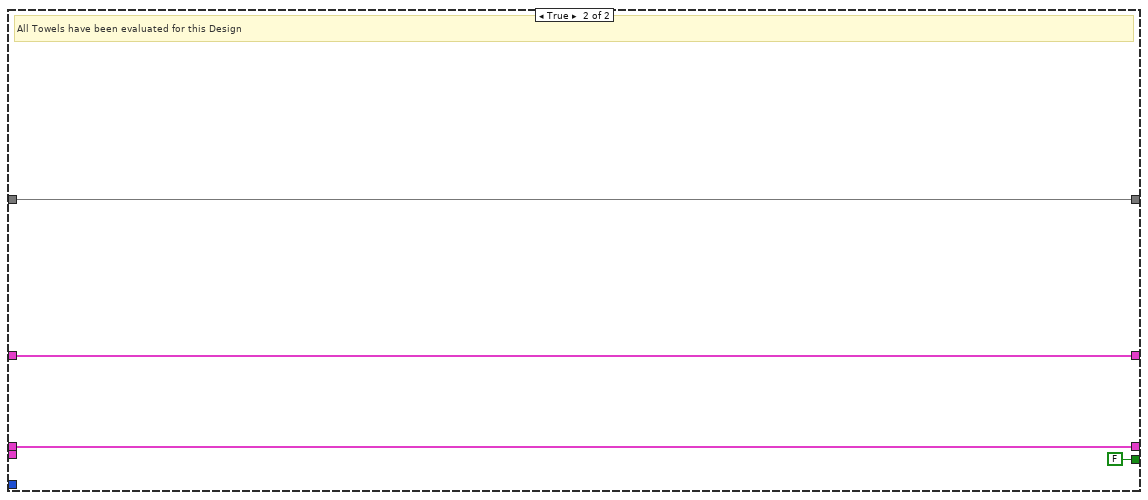
[diagram p5: hidden frame]
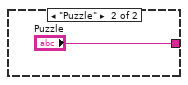
[diagram p6: hidden frame]
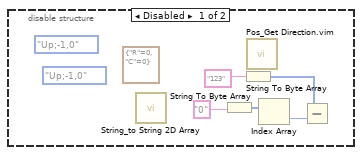
[diagram p7: hidden frame]
diagram:
  w7 = map{i32, i32} {}  # Size: 0
  # "Sort Largest\nto Smallest\nby size"
  n1 = case shown="\"Example\", Default" "Select Data" {
    tunnel: ["Example" "Puzzle"] -> w20
    frame "Example", Default {
    }
    frame "Puzzle" {
    }
  }
  n2 = disable-structure shown="Enabled" {
    frame Disabled {
      (unwired) ENUM_8_Directions_U-D-L-R."Up;-1,0" ("Direction 8")
      (unwired) ENUM_4_Directions_U-D-L-R."Up;-1,0" ("Direction")
      (unwired) T7 {"R"=0, "C"=0} ("Position")
      n3 = call "String_to String 2D Array.vi"() -> ()  [unwired: 11 in, 1 out]
      n4 = String To Byte Array(string="0") -> (unsigned byte array=w28:u8[])
      n5 = String To Byte Array(string="123") -> (unsigned byte array=w26:u8[])
      n6 = call "Pos_Get Direction.vim"() -> ()  [unwired: 11 in, 1 out]
      n7 = Index Array(array=w28) -> (element=w27:u8)  [unwired: 1 in]
      n8 = Subtract(x=w26, y=w27) -> ()  [unwired: 1 out]
    }
    frame Enabled {
    }
  }
  n9 = call <vilib>:"Delimited String to 1D String Array.vi"("delimiter"="\n\n" ("delimiter (Tab)"), "delimited string"=w20) -> ("string array"=w19:string[])  [unwired: 9 in]
  n10 = Index Array(array=w19, index #1=1 ("index"), index #2=0 ("index")) -> (element #1=w8:string, element #2=w9:string)
  n11 = call <vilib>:"Delimited String to 1D String Array.vi"("delimiter"=", " ("delimiter (Tab)"), "delimited string"=w9) -> ("string array"=w16:string[])  [unwired: 9 in]
  n12 = for {
    tunnel: w16 -> [w31] mode=indexing
    tunnel: [w33] -> w15 mode=indexing
    n13 = String Length(string=w31) -> (length=w34:i32)
    n14 = Bundle(cluster=T4 {"Size"=0, "String"="", "ID"=0} ("Stripe Data"), "Size"=w34, "String"=w31) -> (w33:T4)  [unwired: 1 in]
  }
  n15 = call <vilib>:"Delimited String to 1D String Array.vi"("delimiter"="\n" ("delimiter (Tab)"), "delimited string"=w8) -> ("string array"=w14:string[])  [unwired: 9 in]
  "Target Design" <- w14
  n16 = Sort 1D Array(array=w15) -> (sorted array=w13:T4[])
  n17 = Reverse 1D Array(array=w13) -> (reversed array=w4:T4[])
  n18 = for {
    tunnel: w14 -> [w36] mode=indexing
    tunnel: [w37] -> w12 mode=indexing
    i -> [w35]
    n19 = call "Build Design Cluster from String.vi"("Design ID"=w35, "Stripe String"=w36) -> ("Stripe Data"=w37:T1)  [unwired: 9 in]
  }
  n20 = for {
    tunnel: w4 -> [w40] mode=indexing
    tunnel: [w39] -> w3 mode=indexing
    i -> [w38]
    n21 = Bundle By Name(cluster=w40, "ID"=w38) -> (w39:T4)
  }
  "Towel List" <- w3
  n22 = while {
    shift-right: [w57] -> _
    shift-left: w12 -> [w61]
    tunnel: w3 -> [w50]
    shift-right: [w58] -> w6
    shift-left: w7 -> [w45]
    tunnel: [w54] -> w2 mode=indexing if=w53
    tunnel: [w54] -> w1 mode=indexing if=w52
    stop <- w55 stop-if-true
    # "Process Designs until the array is empty"
    n23 = Delete From Array(array=w61, index=0) -> (deleted portion=w46:T1, array with subset deleted=w59:T1[])  [unwired: 1 in]
    n24 = Unbundle By Name(w46) -> ("Last Eval Towel"=w51:i32)
    n25 = Unbundle By Name(w46) -> ("Design ID"=w44:i32)
    n26 = Array Size(array=w50) -> (size(s)=w48:i32)
    n27 = Increment(x=w51) -> (x+1=w49:i32)
    n28 = Look In Map(map=w45, key=w44) -> (key not found?=w43:bool)  [unwired: 1 in, 1 out]
    n29 = Greater Or Equal?(x=w49, y=w48) -> (x >= y?=w47:bool)
    n30 = Not(x=w43) -> (.not. x?=w41:bool)
    n31 = Or(x=w41, y=w47) -> (x .or. y?=w42:bool)
    n32 = case shown="False" w42 {
      tunnel: w59 -> [w71 w120]
      tunnel: w45 -> [w70 w119]
      tunnel: [w69 w119] -> w58
      tunnel: [w68 w120] -> w57
      tunnel: [w67 w122] -> w54
      tunnel: [w66 FALSE] -> w53
      tunnel: w46 -> [w65 w122]
      tunnel: w50 -> [w63 _]
      tunnel: w49 -> [w62 _]
      frame False {
        # "Remove\nPreviously\nEvaluated\nTowels"
        # "Towels Left for Evaluation"
        n33 = Array Subset(array=w63, index=w62) -> (w64:T4[])  [unwired: 1 in]
        n34 = for {
          tunnel: w64 -> [w89] mode=indexing
          shift-right: [w86] -> w68
          shift-left: w71 -> [w87]
          shift-right: [w84] -> w69
          shift-left: w70 -> [w85]
          shift-right: [w83] -> w67
          shift-left: w65 -> [w88]
          tunnel: [w72] -> w66
          stop <- w72 stop-if-true
          # "For Each Towel"
          n35 = call "Search and Match Towel to Design.vi"("Towel"=w89, "Design Data"=w88) -> ("Check If Full Out"=w73:bool, "Design Array Out"=w80:T1[])  [unwired: 8 in]
          "Design Updated" <- w73
          n36 = Split 1D Array(array=w80, index=1) -> (first subarray=w78:T1[], second subarray=w75:T1[])
          n37 = Build Array (concatenate)(w75, w87) -> (w76:T1[])
          n38 = Index Array(array=w78, index=0) -> (element=w82:T1)
          "New Design" <- w82
          n39 = case shown="False" w73 {
            tunnel: w82 -> [w90 w91]
            tunnel: [_ w92] -> w81
            tunnel: [w90 w91] -> w74
            frame False {
            }
            frame True {
              n40 = call "Check Design Array Full.vi"("Design Data"=w91) -> ("Design Array Full"=w92:bool)  [unwired: 10 in]
            }
          }
          n41 = case shown="True" w81 {
            selector: w81 -> [_ w97]
            tunnel: w74 -> [w93 w96]
            tunnel: w76 -> [w94 w105]
            tunnel: [w94 w105] -> w86
            tunnel: w85 -> [w95 w104]
            tunnel: [w95 w103] -> w84
            tunnel: [_ w97] -> w72
            tunnel: [w93 w96] -> w83
            frame False {
              # "Design is Not Full"
            }
            frame True {
              w101 = set{i32} {}  # Size: 0
              # "Design is Full"
              n42 = Unbundle By Name(w96) -> ("Design ID"=w102:i32)
              n43 = Unbundle By Name(w96) -> ("T-Array"=w100:T3[])
              n44 = for {
                shift-right: [w107] -> w99
                shift-left: w101 -> [w108]
                tunnel: w100 -> [w109] mode=indexing
                n45 = Unbundle By Name(w109) -> ("Start Index"=w106:i32)
                n46 = Insert Into Set(10:w106, 11:w108) -> (3:w107:set{i32})  [unwired: 1 out]
              }
              n47 = Collection Size(1:w99) -> (0:w98:i32)
              n48 = in-place {
                in-place-border: w98 -> [w113]
                n49 = in-place-map #1(w104, w102) -> (w114:i32, w110:bool)  [unwired: 1 in]
                n50 = case shown="False" w110 {
                  tunnel: w114 -> [w117 _]
                  tunnel: w113 -> [w116 w118]
                  tunnel: [w115 w118] -> w112
                  frame False {
                    # "keep smallest"
                    # "Key Present"
                    n51 = Max & Min(x=w117, y=w116) -> (min(x,y)=w115:i32)  [unwired: 1 out]
                  }
                  frame True {
                    # "New Key"
                  }
                }
                n52 = in-place-map #1(w112, LVMapReplaceAction."Add or Modify Entry" ("action")) -> (w103:map{i32, i32})  [unwired: 2 out]
              }
            }
          }
          "Current Design" <- w88
          "Current Towel" <- w89
        }
      }
      frame True {
        # "All Towels have been evaluated for this Design"
      }
    }
    n53 = Array Size(array=w57) -> (size(s)=w56:i32)
    n54 = Not(x=w53) -> (.not. x?=w52:bool)
    n55 = Less Or Equal To 0?(x=w56) -> (x <= 0?=w55:bool)
  }
  "Valid Designs" <- w2
  "Invalid Designs" <- w1
  n56 = Collection Size(1:w6) -> (0:w5:i32)
  n57 = To Unsigned Long Integer(number=w5) -> (unsigned 32bit integer=→"Answer":u32)
